vi "Set Lighting all Devices.vi"(8 "error in (no error)":errorcluster, 11 "LED Color":u32(colorbox)) -> (0 "error out":errorcluster)   [LabVIEW 2022 SP3, in "Logitech Devices.lvlib"]
uses:
  Logitech Devices.lvlib
  C:/Program Files/LGHUB/sdks/sdk_legacy_led_x86.dll
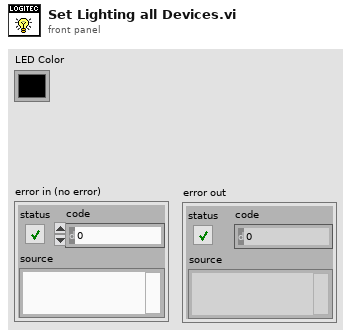
[diagram p1: front panel]
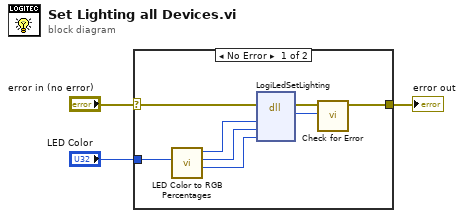
[diagram p0: block diagram]
diagram:
  n1 = case shown="No Error" "error in (no error)" {
    selector: "error in (no error)" -> [w11 w12]
    tunnel: [w4 w12] -> w2
    tunnel: "LED Color" -> [w9 _]
    frame No Error {
      n2 = call "LED Color to RGB Percentages.vi"("LED Color"=w9) -> ("Blue %"=w6:u8, "Green %"=w7:u8, "Red %"=w8:u8)  [unwired: 8 in]
      n3 = dll-call lib="C:/Program Files/LGHUB/sdks/sdk_legacy_led_x86.dll" fn="LogiLedSetLighting"(error in=w11, "Red Percentage"=w8, "Green Percentage"=w7, "Blue Percentage"=w6) -> (error out=w5:errorcluster, "return type"=w10:u8)  [unwired: 5 in, 1 out]
      n4 = call "Check for Error.vi"("DLL-call return value"=w10, "error in (no error)"=w5) -> ("error out"=w4:errorcluster)  [unwired: 9 in]
    }
    frame Error {
    }
  }
  "error out" <- w2
